vi "Evaluate Part 2_rev2.vi"() -> ()   [LabVIEW 2020]
uses:
  Range/Range.lvclass
  Map/Map.lvclass
  Range Map/Range Map.lvclass
panel:
  out "min value":u32
  in  "Input":string="seeds: 79 14 55 13\n\nseed-to-soil map:\n50 98 2\n52 50 48\n\nsoil-to-fertilizer map:\n0 15 37\n37 52 2\n39 0 15\n\nfertilizer-to-water map:\n49 53 8\n0 11 42\n42 0 7\n57 7 4\n\nwater-to-light map:\n88 18 7\n18 25 70\n\nlight-to-temperature map:\n45 77 23\n81 45 19\n68 64 13\n\ntemperature-to-humidity map:\n0 69 1\n1 0 69\n\nhumidity-to-location map:\n60 56 37\n56 93 4"
  # "20283860"
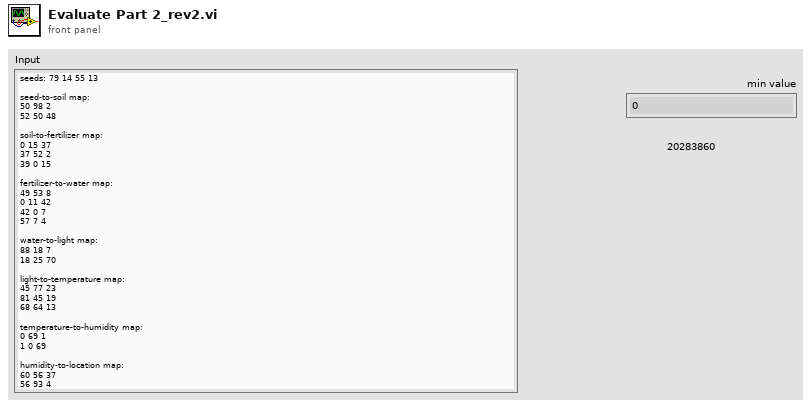
[diagram p1: front panel]
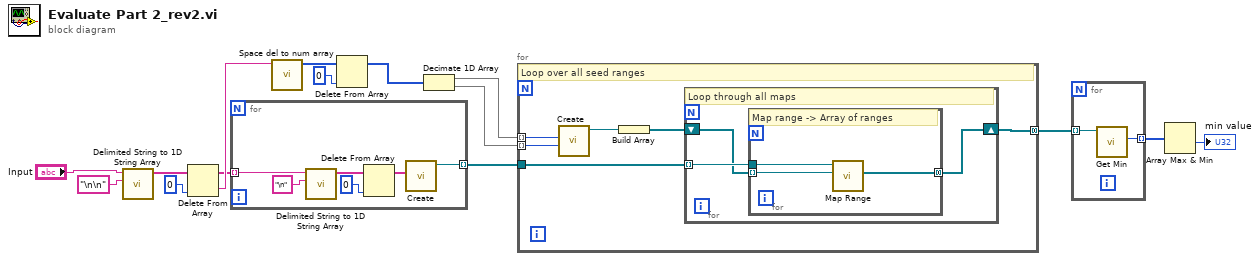
[diagram p0: block diagram]
diagram:
  n1 = call <vilib>:"Delimited String to 1D String Array.vi"("delimiter"="\n\n" ("String"), "delimited string"="Input") -> ("string array"=w10:string[])  [unwired: 9 in]
  n2 = Delete From Array(array=w10, index=0) -> (deleted portion=w13:string, array with subset deleted=w9:string[])  [unwired: 1 in]
  n3 = for {
    tunnel: w9 -> [w19] mode=indexing
    tunnel: [w16] -> w5 mode=indexing
    n4 = call <vilib>:"Delimited String to 1D String Array.vi"("delimiter"="\n" ("String"), "delimited string"=w19) -> ("string array"=w18:string[])  [unwired: 9 in]
    n5 = Delete From Array(array=w18, index=0) -> (array with subset deleted=w17:string[])  [unwired: 1 in, 1 out]
    n6 = call "Create.vi"("Input"=w17) -> ("Range Map"=w16:refnum<class "Range Map.lvclass">)  [unwired: 9 in, 1 out]
  }
  n7 = call "Space del to num array.vi"("Input in"=w13) -> ("Input out"=w12:u64[])  [unwired: 10 in]
  n8 = Delete From Array(array=w12, index=0) -> (array with subset deleted=w8:u64[])  [unwired: 1 in, 1 out]
  n9 = Decimate 1D Array(w8) -> (w7:u64[], w6:u64[])
  n10 = for {
    tunnel: w5 -> [w27]
    tunnel: w7 -> [w24] mode=indexing
    tunnel: w6 -> [w23] mode=indexing
    tunnel: [w22] -> w4 mode=concatenating
    # "Loop over all seed ranges"
    n11 = call "Create.vi"("Length"=w23, "From"=w24) -> ("Range"=w26:refnum<class "Range.lvclass">)  [unwired: 8 in, 1 out]
    n12 = Build Array(w26) -> (w25:refnum<class "Range.lvclass">[])
    n13 = for {
      tunnel: w27 -> [w30] mode=indexing
      shift-right: [w28] -> w22
      shift-left: w25 -> [w29]
      # "Loop through all maps"
      n14 = for {
        tunnel: w30 -> [w33]
        tunnel: w29 -> [w32] mode=indexing
        tunnel: [w31] -> w28 mode=concatenating
        # "Map range -> Array of ranges"
        n15 = call "Map Range.vi"("Range"=w32, "Range Map in"=w33) -> ("Ranges"=w31:refnum<class "Range.lvclass">[])  [unwired: 7 in, 2 out]
      }
    }
  }
  n16 = for {
    tunnel: w4 -> [w35] mode=indexing
    tunnel: [w34] -> w3 mode=indexing
    n17 = call "Get Min.vi"("Range in"=w35) -> ("Min"=w34:u64)  [unwired: 8 in, 2 out]
  }
  n18 = Array Max & Min(array=w3) -> (min value=→"min value":u64)  [unwired: 3 out]
